vi "float_switch_check.vi"(0 "Temperature Refnum":refnum<vi>, 1 "Heater Refnum":refnum<vi>, 2 "Abs Pressure Refnum":refnum<vi>, 3 "InvertLines":bool, 4 "Abs Temperature Limit Refnum":refnum<vi>, 5 "Timeout Refnum":refnum<vi>, 6 "Abs Pressure Limit Refnum":refnum<vi>, 7 "STOP! Refnum":refnum<vi>, 8 "Pulse Generator Slide Refnum":refnum<vi>, 9 "Float Indicator Refnum":refnum<vi>[](array[refnum]), 10 "lines array":tag[](array[tag])) -> ()   [LabVIEW 2017]
doc: "Continuously monitor the Pulse Generator float valves' status, absolute pressure and temperature. Each reading is used to determine if the pulse generator fluid is at a safe state. Excess or insufficient liquid will trigger the display of warning signs on the main front panel. Excess pressure and temperature will shuts off the pulse generator heaters."
uses:
  <vilib>/DAQmx/read.llb/DAQmx Read (Digital 1D Bool NChan 1Samp 1Line).vi
  <vilib>/DAQmx/create/channels.llb/DAQmx Create Channel (DI-Digital Input).vi
  <vilib>/DAQmx/miscellaneous.llb/DAQmx Fill In Error Info.vi
  <resource>/objmgr/daqmx.rc
panel:
  out "Numeric":i32
  out "Stopwatch Elapsed":dbl
  out "Stopwatch Start":dbl
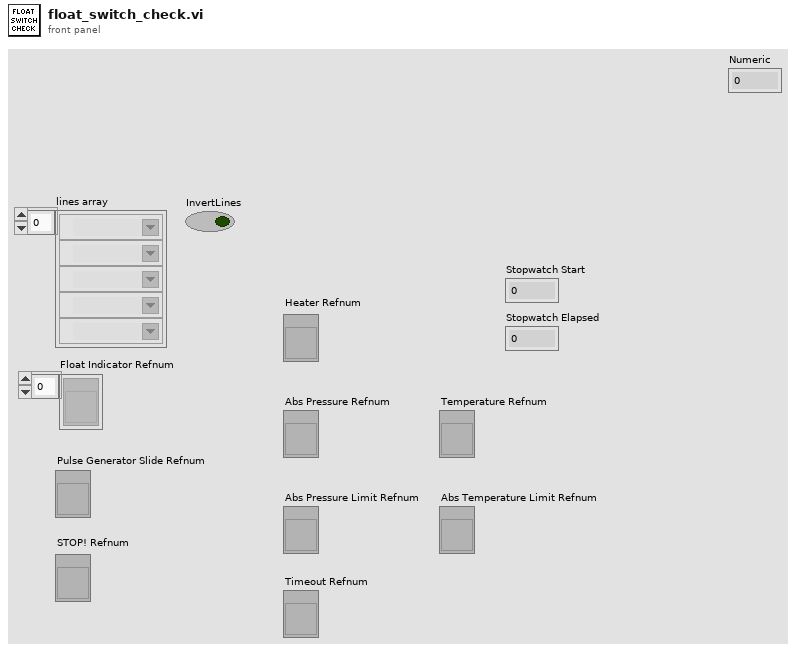
[diagram p1: front panel]
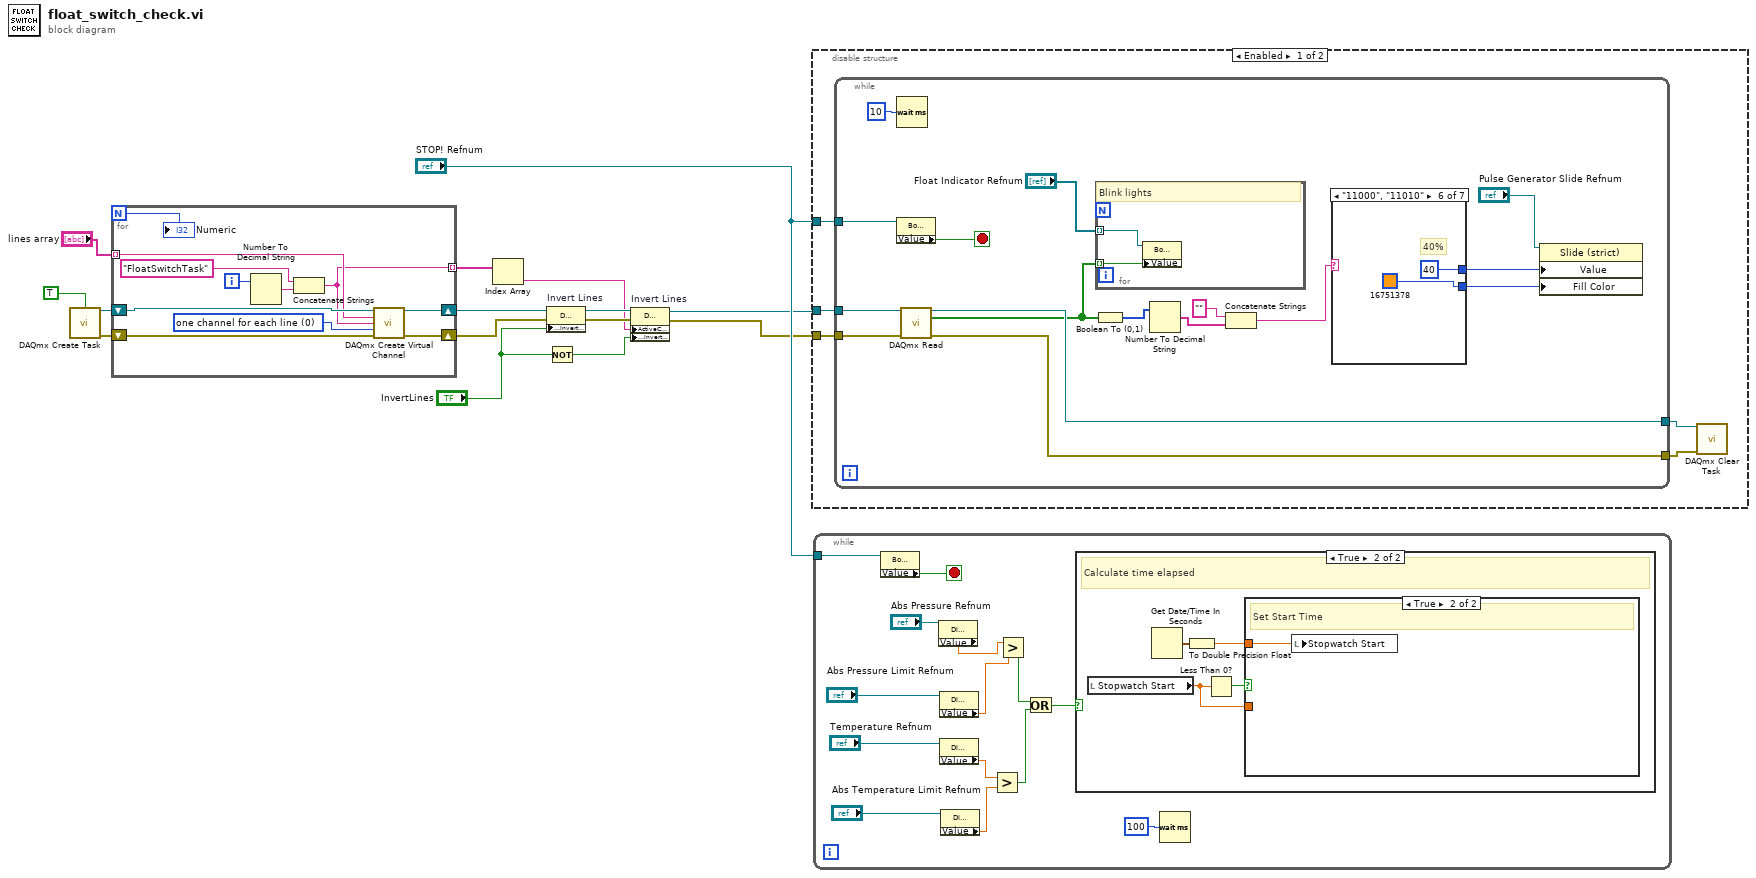
[diagram p0: block diagram]
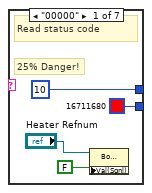
[diagram p2: hidden frame]
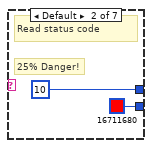
[diagram p3: hidden frame]
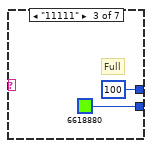
[diagram p4: hidden frame]
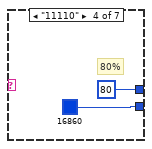
[diagram p5: hidden frame]
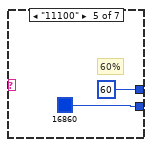
[diagram p6: hidden frame]
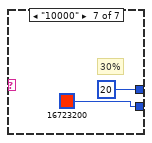
[diagram p7: hidden frame]
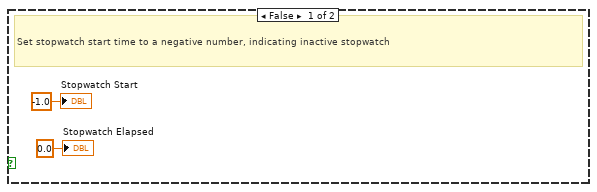
[diagram p9: hidden frame]
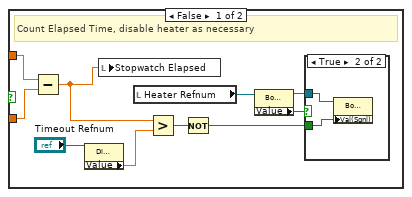
[diagram p10: hidden frame]
diagram:
  n1 = call <vilib>:"DAQmx Create Task.vi"("auto cleanup"=TRUE) -> ("task out"=w14:refnum<k21>, "error out"=w13:errorcluster)  [unwired: 13 in]
  n2 = for {
    N -> [w18]
    shift-right: [w26] -> w11
    shift-left: w14 -> [w24]
    shift-right: [w25] -> w10
    shift-left: w13 -> [w23]
    tunnel: "lines array" -> [w22] mode=indexing
    tunnel: [w16] -> w2 mode=indexing
    i -> [w19]
    w20 = 0 items=["one channel for each line", "one channel for all lines"] ("line grouping")
    n3 = Number To Decimal String(number=w19) -> (decimal integer string=w21:string)  [unwired: 1 in]
    n4 = Concatenate Strings("FloatSwitchTask" ("string"), w21) -> (w16:string)
    n5 = call-poly <vilib>:"DAQmx Create Virtual Channel.vi"("task in"=w24, "lines"=w22, "name to assign"=w16, "line grouping"=w20, "error in"=w23) -> ("task out"=w26:refnum<k21>, "error out"=w25:errorcluster)  [unwired: 9 in]
    "Numeric" <- w18
  }
  n6 = Index Array(array=w2) -> (element=w1:string)  [unwired: 1 in]
  n7 = property on="Invert Lines" class="DAQmx Channel"(reference=w11, error in=w10, "DI.InvertLines"="InvertLines") -> (reference out=w8:refnum<k21>, error out=w7:errorcluster)
  n8 = Not(x="InvertLines") -> (.not. x?=w3:bool)
  n9 = property on="Invert Lines" class="DAQmx Channel"(reference=w8, error in=w7, "ActiveChans"=w1, "DI.InvertLines"=w3) -> (reference out=w6:refnum<k21>, error out=w5:errorcluster)
  n10 = disable-structure shown="Enabled" {
    disable-tunnel: w6 -> [w31 _]
    disable-tunnel: w5 -> [w30 _]
    disable-tunnel: "STOP! Refnum" -> [w27 _]
    frame Enabled {
      n11 = while {
        tunnel: w31 -> [w45]
        tunnel: w30 -> [w44]
        tunnel: w27 -> [w40]
        tunnel: [w38] -> w29
        tunnel: [w37] -> w28
        stop <- w39 stop-if-true
        n12 = Wait (ms)(milliseconds to wait=u32 10) -> ()  [unwired: 1 out]
        n13 = property class="Bool (strict)"(reference=w40) -> ("Value"=w39:bool)  [unwired: 1 in, 2 out]
        n14 = call-poly <vilib>:"DAQmx Read.vi"("task/channels in"=w45, "error in"=w44) -> ("task out"=w38:refnum<k21>, "data"=w36:bool[], "error out"=w37:errorcluster)  [unwired: 11 in]
        n15 = Boolean To (0,1)(Boolean=w36) -> (0, 1=w35:i16[])
        n16 = for {
          tunnel: w36 -> [w65] mode=indexing
          tunnel: "Float Indicator Refnum" -> [w64] mode=indexing
          # "Blink lights"
          n17 = property class="Bool (strict)"(reference=w64, "Value"=w65) -> ()  [unwired: 1 in, 2 out]
        }
        n18 = Number To Decimal String(number=w35) -> (decimal integer string=w34:string[])  [unwired: 1 in]
        n19 = Concatenate Strings("" ("string"), w34) -> (w32:string)
        n20 = case shown="\"11000\", \"11010\"" w32 {
          tunnel: [u8 10 u8 10 u8 100 u8 80 u8 60 u8 40 u8 20] -> w47
          tunnel: [u32 16711680 u32 16711680 u32 6618880 u32 16860 u32 16860 u32 16751378 u32 16723200] -> w46
          frame "00000" {
            # "25% Danger!"
            # "Read status code"
            n21 = property class="Bool (strict)"(reference="Heater Refnum", "Val(Sgnl)"=FALSE) -> ()  [unwired: 1 in, 2 out]
          }
          frame Default {
            # "25% Danger!"
            # "Read status code"
          }
          frame "11111" {
            # "Full"
          }
          frame "11110" {
            # "80%"
          }
          frame "11100" {
            # "60%"
          }
          frame "11000", "11010" {
            # "40%"
          }
          frame "10000" {
            # "30%"
          }
        }
        n22 = property class="Slide (strict)"(reference="Pulse Generator Slide Refnum", "Value"=w47, "Fill Color"=w46) -> ()  [unwired: 1 in, 2 out]
      }
      n23 = call <vilib>:"DAQmx Clear Task.vi"("task in"=w29, "error in"=w28) -> ()  [unwired: 13 in, 1 out]
    }
    frame Disabled {
    }
  }
  n24 = while {
    tunnel: "STOP! Refnum" -> [w78]
    stop <- w79 stop-if-true
    n25 = property class="Bool (strict)"(reference=w78) -> ("Value"=w79:bool)  [unwired: 1 in, 2 out]
    n26 = property class="DigNum (strict)"(reference="Abs Pressure Refnum") -> ("Value"=w67:dbl)  [unwired: 1 in, 2 out]
    n27 = property class="DigNum (strict)"(reference="Abs Pressure Limit Refnum") -> ("Value"=w66:dbl)  [unwired: 1 in, 2 out]
    n28 = property class="DigNum (strict)"(reference="Temperature Refnum") -> ("Value"=w72:dbl)  [unwired: 1 in, 2 out]
    n29 = property class="DigNum (strict)"(reference="Abs Temperature Limit Refnum") -> ("Value"=w71:dbl)  [unwired: 1 in, 2 out]
    n30 = Greater?(x=w72, y=w71) -> (0:w69:bool)
    n31 = Greater?(x=w67, y=w66) -> (0:w70:bool)
    n32 = Or(x=w70, y=w69) -> (x .or. y?=w68:bool)
    n33 = case shown="True" w68 {
      frame False {
        # "Set stopwatch start time to a negative number, indicating inactive stopwatch"
        "Stopwatch Start" <- -1.0 ("Stopwatch Start")
        "Stopwatch Elapsed" <- 0.0 ("Stopwatch Elapsed")
      }
      frame True {
        # "Calculate time elapsed"
        n34 = local read "Stopwatch Start"() -> (w82:dbl)
        n35 = Get Date/Time In Seconds() -> (seconds since 1Jan1904=w84:timestamp)
        n36 = To Double Precision Float(number=w84) -> (double precision float=w83:dbl)
        n37 = Less Than 0?(x=w82) -> (x < 0?=w85:bool)
        n38 = case shown="True" w85 {
          tunnel: w83 -> [w95 w98]
          tunnel: w82 -> [w94 _]
          frame False {
            # "Count Elapsed Time, disable heater as necessary"
            n39 = Subtract(x=w95, y=w94) -> (x-y=w90:dbl)
            n40 = property class="DigNum (strict)"(reference="Timeout Refnum") -> ("Value"=w92:dbl)  [unwired: 1 in, 2 out]
            n41 = local write "Stopwatch Elapsed"(w90) -> ()
            n42 = local read "Heater Refnum"() -> (w89:refnum<vi>)
            n43 = Greater?(x=w90, y=w92) -> (0:w91:bool)
            n44 = Not(x=w91) -> (.not. x?=w86:bool)
            n45 = property class="Bool (strict)"(reference=w89) -> (reference out=w87:refnum<vi>, "Value"=w88:bool)  [unwired: 1 in, 1 out]
            n46 = case shown="True" w88 {
              tunnel: w87 -> [_ w97]
              tunnel: w86 -> [_ w96]
              frame False {
              }
              frame True {
                n47 = property class="Bool (strict)"(reference=w97, "Val(Sgnl)"=w96) -> ()  [unwired: 1 in, 2 out]
              }
            }
          }
          frame True {
            # "Set Start Time"
            n48 = local write "Stopwatch Start"(w98) -> ()
          }
        }
      }
    }
    n49 = Wait (ms)(milliseconds to wait=u32 100) -> ()  [unwired: 1 out]
  }
